vi "HW1.vi"() -> ()   [LabVIEW 2020]
panel:
  out "Array 2":dbl[](array[numeric])
  out "Numeric 2":dbl
  out "Array":i32[](array[numeric])
  out "Numeric":i32
  out "x+1":i32
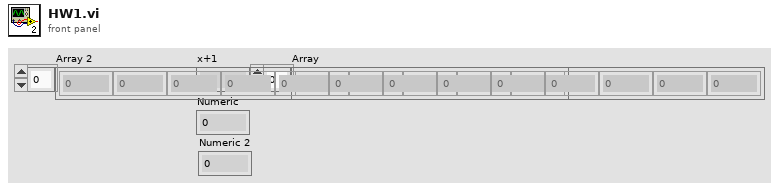
[diagram p1: front panel]
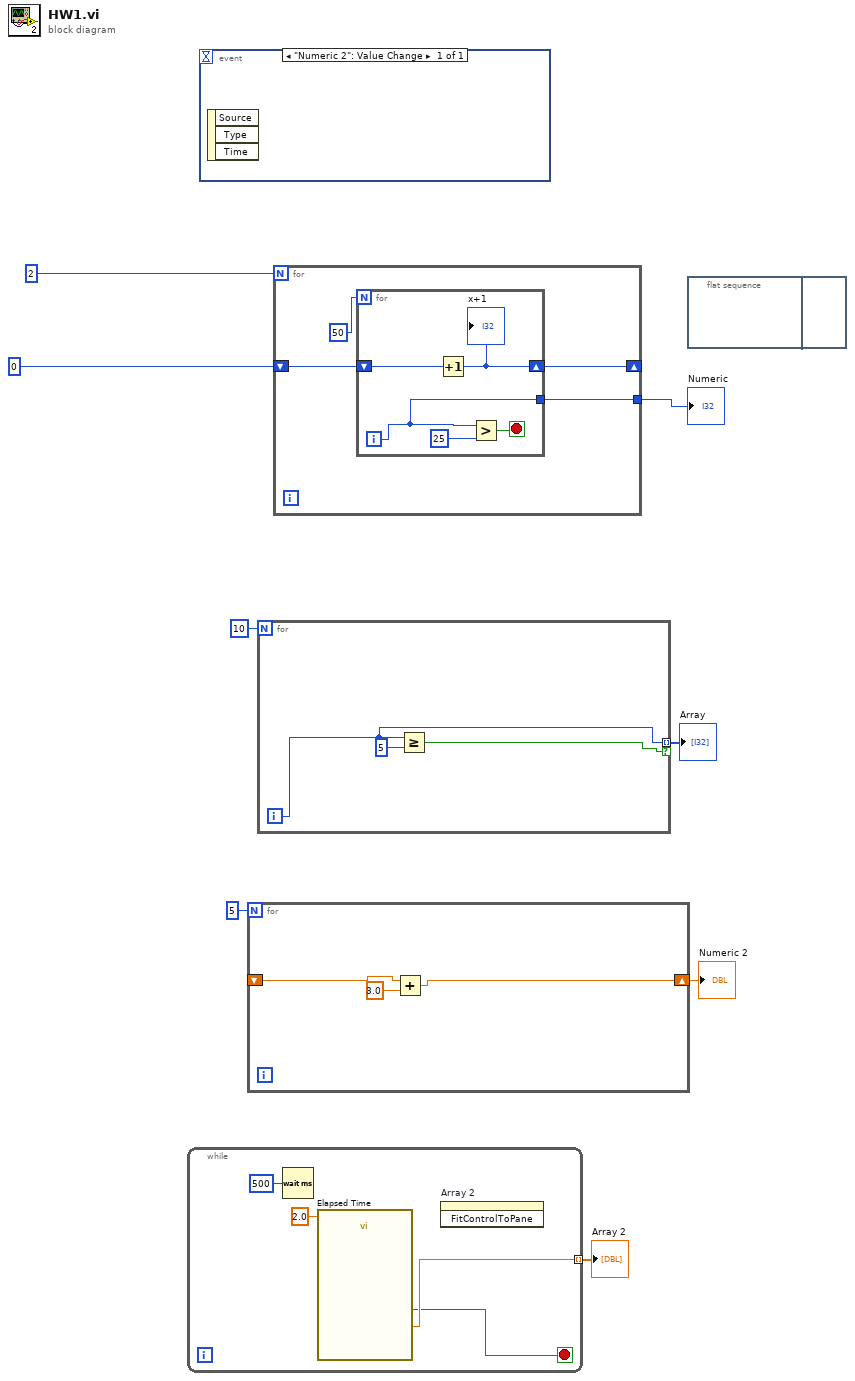
[diagram p0: block diagram]
diagram:
  n1 = while {
    tunnel: [w10] -> w1 mode=indexing
    stop <- w9 stop-if-true
    n2 = Wait (ms)(milliseconds to wait=u32 500) -> ()  [unwired: 1 out]
    n3 = call "Elapsed Time"("Time Target (s)"=2.0) -> ("Elapsed Time (s)"=w10:dbl, "Time has Elapsed"=w9:bool)  [unwired: 11 in, 6 out]
    n4 = invoke on="Array 2" class="Arr (strict)" method="FitControlToPane"() -> ()  [unwired: 3 in, 3 out]
  }
  "Array 2" <- w1
  n5 = event shown="[0] \"Numeric 2\": Value Change" {
    selector: _ -> [_]
    dyn-events: _ -> [_]
    timeout: _ -> [_]
    event "Numeric 2": Value Change {
      n6 = event-data() -> ()  [unwired: 1 in, 3 out]
    }
  }
  n7 = for {
    N: 5 -> [_]
    shift-right: [w13] -> w2
    shift-left: _ -> [w14]
    n8 = Add(x=w14, y=3.0) -> (x+y=w13:dbl)
  }
  "Numeric 2" <- w2
  n9 = for {
    N: 10 -> [_]
    tunnel: [w16] -> w4 mode=indexing if=w17
    i -> [w16]
    n10 = Greater Or Equal?(x=w16, y=5) -> (x >= y?=w17:bool)
  }
  "Array" <- w4
  n11 = for {
    N: 2 -> [_]
    shift-right: [w22] -> _
    shift-left: 0 -> [w21]
    tunnel: [w19] -> w6
    n12 = for {
      N: 50 -> [_]
      shift-right: [w25] -> w22
      shift-left: w21 -> [w26]
      tunnel: [w23] -> w19
      i -> [w23]
      stop <- w24 stop-if-true
      n13 = Increment(x=w26) -> (x+1=w25:i32)
      "x+1" <- w25
      n14 = Greater?(x=w23, y=25) -> (0:w24:bool)
    }
  }
  "Numeric" <- w6
  n15 = flat-sequence {
    frame #0 {
    }
    frame #1 {
    }
  }
